vi "UpdateGlobals.vi"(0 "error in (no error)":errorcluster, 2 "Operator Listbox Ref":refnum<vi>, 3 "Doctor Listbox Ref":refnum<vi>) -> (7 "error out":errorcluster)   [LabVIEW 2013, in "main.lvlib"]
uses:
  main.lvlib
  Controls/Enum Save Action Events.ctl
  Controls/Enum Globals.ctl
  Controls/Enum Variables.ctl
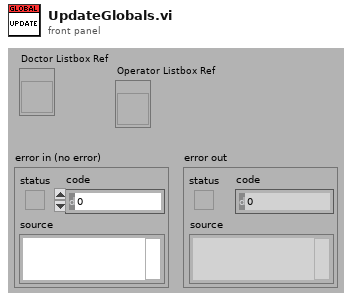
[diagram p1: front panel]
types:
  T1 = typedef "main.lvlib/Enum Save Action Events.ctl" = enum16{"LoadReportPath", "SaveReportPath", "Load Graph Path", "Save Graph Path", "LoadDataPath", "SaveDataPath", "Load Template Path", "Save Template Path", "Load PressureFactor", "Save PressureFactor", "Init", "Load Listbox", "Save Listbox", "LoadHospInfo", "SaveHospInfo", "Load DICOM Activation", "Save DICOM Activation", "LoadDICOMInfoWL", "SaveDICOMInfoWL", "LoadDICOMInfoPACS", "SaveDICOMInfoPACS", "Load ArmCalcMethod", "Save ArmCalcMethod", "LoadItemTags", "SaveItemTags", "LoadDICOMEncoding", "SaveDICOMEncoding", "LoadJournalType", "SaveJournalType", "LoadAcqFilterType", "SaveAcqFilterType", "Load Sequence", "Save Sequence", "Load Acquisition Mode", "Save Acquisition Mode", "Load General Settings", "Save General Settings", "Load Language", "Save Language", "Load Dicom Tags", "Save Dicom Tags", "Load BT Serial", "Save BT Serial", "Load BT License", "Save BT License"}
  T2 = typedef "main.lvlib/Enum Variables.ctl" = enum16{"SetAcqFilter", "GetAcqFilter", "Set Filter", "Get Filter", "Set Height", "Get Height", "Set Recorded Height", "Get Recorded Height", "Set Blue Pressure", "Get Blue Pressure", "Set Red Pressure", "Get Red Pressure", "Init", "Reset Pressure", "Set Red Cursors", "Get Red Cursors", "Set Blue Cursors", "Get Blue Cursors", "Set Language", "Get Language", "Set Active Graphs", "Get ActiveGraphs", "Set Method", "Get Method", "Set Encryption", "Get Encryption", "Set ExcelVersion", "Get ExcelVersion", "Set DICOM Avail", "Get DICOM Avail", "Set DICOM Encode", "Get DICOM Encode", "Set JournalExport", "Get JournalExport", "Set Sequence", "Get Sequence", "Set DAQ Connected", "Get DAQ Connected", "Set Current Graph", "Get Current Graph", "Set General Settings", "Get Hyphenation", "Set Arm Calc Method", "Get Arm Calc Method", "Set Dicom Tags", "Get Dicom Tags", "Set BT Serial", "Get BT Serial", "Set BT Accepted Serials", "Get BT Accepted Serials", "Get BT License", "Set BT License"}
  T3 = typedef "main.lvlib/Enum Globals.ctl" = enum16{"Init", "Set DataPath", "Set Freq", "Get"}
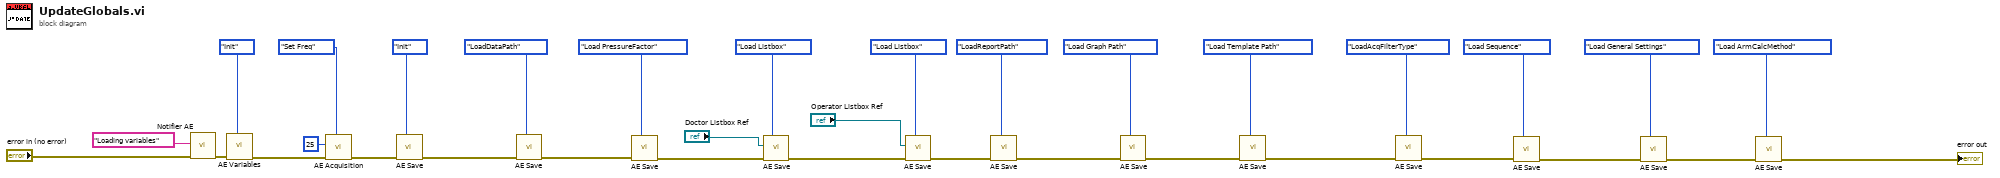
[diagram p0: block diagram]
diagram:
  n1 = call "Notifier AE.vi"("error in (no error)"="error in (no error)", "String"="Loading variables") -> ("error out"=w10:errorcluster)  [unwired: 9 in]
  n2 = call "AE Variables.vi"("error in (no error)"=w10, "Action"=Enum_Variables."Init") -> ("error out"=w17:errorcluster)  [unwired: 10 in, 7 out]
  n3 = call "AE Acquisition.vi"("Action"=Enum_Globals."Set Freq", "error in (no error)"=w17, "Freq"=25) -> ("error out"=w22:errorcluster)  [unwired: 5 in, 3 out]
  n4 = call "AE Save.vi"("error in (no error)"=w22, "Action"=Enum_Save_Action_Events."Init") -> ("error out"=w21:errorcluster)  [unwired: 7 in, 1 out]
  n5 = call "AE Save.vi"("error in (no error)"=w21, "Action"=Enum_Save_Action_Events."LoadDataPath") -> ("error out"=w27:errorcluster)  [unwired: 7 in, 1 out]
  n6 = call "AE Save.vi"("error in (no error)"=w27, "Action"=Enum_Save_Action_Events."Load PressureFactor") -> ("error out"=w33:errorcluster)  [unwired: 7 in, 1 out]
  n7 = call "AE Save.vi"("error in (no error)"=w33, "LstBox Refnum"="Doctor Listbox Ref", "Action"=Enum_Save_Action_Events."Load Listbox") -> ("error out"=w31:errorcluster)  [unwired: 6 in, 1 out]
  n8 = call "AE Save.vi"("error in (no error)"=w31, "LstBox Refnum"="Operator Listbox Ref", "Action"=Enum_Save_Action_Events."Load Listbox") -> ("error out"=w1:errorcluster)  [unwired: 6 in, 1 out]
  n9 = call "AE Save.vi"("error in (no error)"=w1, "Action"=Enum_Save_Action_Events."LoadReportPath") -> ("error out"=w14:errorcluster)  [unwired: 7 in, 1 out]
  n10 = call "AE Save.vi"("error in (no error)"=w14, "Action"=Enum_Save_Action_Events."Load Graph Path") -> ("error out"=w2:errorcluster)  [unwired: 7 in, 1 out]
  n11 = call "AE Save.vi"("error in (no error)"=w2, "Action"=Enum_Save_Action_Events."Load Template Path") -> ("error out"=w3:errorcluster)  [unwired: 7 in, 1 out]
  n12 = call "AE Save.vi"("error in (no error)"=w3, "Action"=Enum_Save_Action_Events."LoadAcqFilterType") -> ("error out"=w16:errorcluster)  [unwired: 7 in, 1 out]
  n13 = call "AE Save.vi"("error in (no error)"=w16, "Action"=Enum_Save_Action_Events."Load Sequence") -> ("error out"=w8:errorcluster)  [unwired: 7 in, 1 out]
  n14 = call "AE Save.vi"("error in (no error)"=w8, "Action"=Enum_Save_Action_Events."Load General Settings") -> ("error out"=w7:errorcluster)  [unwired: 7 in, 1 out]
  n15 = call "AE Save.vi"("error in (no error)"=w7, "Action"=Enum_Save_Action_Events."Load ArmCalcMethod") -> ("error out"=→"error out":errorcluster)  [unwired: 7 in, 1 out]
